vi "DAQ_AI_Open.vi"(0 "reference in":refnum<class "NI_DAQ.lvclass">, 5 "error in (no error)":errorcluster) -> (14 "reference out":refnum<class "NI_DAQ.lvclass">, 19 "error out":errorcluster)   [LabVIEW 2020, in "DAQ.lvlib" / "NI_DAQ.lvclass"]
uses:
  NI_DAQ.lvclass
panel:
  out "DAQ_AI_task_out":refnum<k21>
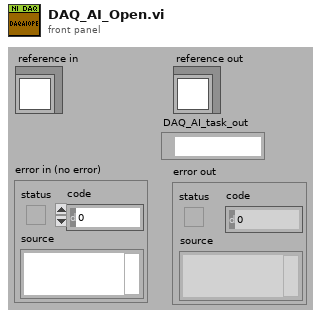
[diagram p1: front panel]
types:
  T1 = typedef "DAQ.lvlib/DAQ_Base.lvclass/DAQSettings.ctl" = cluster{"SampleSettings":T2, "AI_ChannelSettings":T3, "AO_ChannelSettings":T5, "Cnt_ChannelSettings":T6}
  T2 = typedef "DAQ.lvlib/DAQ_Base.lvclass/SampleSettings.ctl" = cluster{"samples per channel":i32, "SampleRate":dbl, "TansMaxLength":dbl, "ReadTimeOut":dbl, "时钟源":tag}
  T3 = typedef "DAQ.lvlib/DAQ_Base.lvclass/AI_ChannelSettings.ctl" = cluster{"AI_SettingsArry":cluster{"DeviceName":tag, "physical channels":tag, "AssignName":string, "输入信号类型":T4, "Max_value":dbl, "Min_value":dbl, "单位":i32, "shunt resistor location":i32, "external shunt resistor value":dbl, "标定系数":cluster{"Scale":dbl, "Offset":dbl}}[]}
  T4 = typedef "AI信号类型.ctl" = i32
  T5 = typedef "DAQ.lvlib/DAQ_Base.lvclass/AO_ChannelSettings.ctl" = cluster{"布尔":bool}
  T6 = typedef "DAQ.lvlib/DAQ_Base.lvclass/Cnt_ChannelSettings.ctl" = cluster{"Cnt_ChannelSettings":cluster{"类型":enum16{"Linear", "Rotate"}, "CounterNbr":tag, "AssignName":string, "单位":u16, "decoding type":u16, "PPR_DistancePerPulse":dbl, "Initial Position ":dbl, "z index enable":bool, "z index phase":i32, "source":tag}[]}
  T7 = typedef "DAQ.lvlib/NI_DAQ.lvclass/ObjectAttributesRef.ctl" = refnum<data-value>
  T8 = typedef "DAQ.lvlib/NI_DAQ.lvclass/ObjectAttributes.ctl" = cluster{"MyAttribute":dbl, "DAQ_AI_task_out":refnum<k21>, "counter_task_out":refnum<k21>[]}
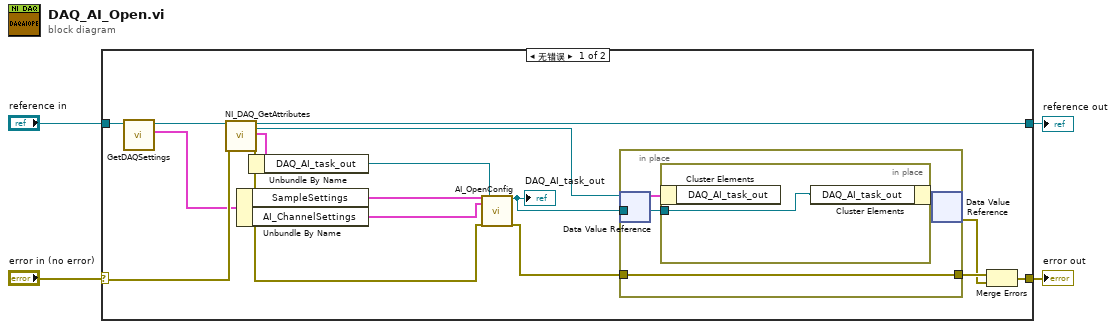
[diagram p0: block diagram]
diagram:
  n1 = case shown="无错误" "error in (no error)" {
    selector: "error in (no error)" -> [w18 w27]
    tunnel: [w20 w27] -> w3
    tunnel: [w19 w26] -> w1
    tunnel: "reference in" -> [w13 w26]
    frame No Error {
      n2 = call-dynamic "GetDAQSettings.vi"("reference in"=w13) -> ("DAQSettings"=w11:T1, "reference out"=w12:refnum<class "NI_DAQ.lvclass">)  [unwired: 8 in, 1 out]
      n3 = call "NI_DAQ_GetAttributes.vi"("reference in"=w12, "error in (no error)"=w18) -> ("reference out"=w19:refnum<class "NI_DAQ.lvclass">, "attributes ref"=w14:T7, "attributes"=w17:T8, "error out"=w9:errorcluster)  [unwired: 14 in]
      n4 = Unbundle By Name(w11) -> ("SampleSettings"=w10:T2, "AI_ChannelSettings"=w6:T3)
      n5 = Unbundle By Name(w17) -> ("DAQ_AI_task_out"=w5:refnum<k21>)
      n6 = call "AI_OpenConfig.vi"("SampleSettings"=w10, "AI_ChannelSettings"=w6, "error in"=w9, "DAQ_AI_task_out"=w5) -> ("DAQ_AI_task_out"=w7:refnum<k21>, "error out"=w8:errorcluster)  [unwired: 14 in]
      "DAQ_AI_task_out" <- w7
      n7 = in-place {
        in-place-border: w8 -> [w22]
        in-place-border: [w22] -> w16
        in-place-border: w7 -> [w21]
        n8 = in-place-dvr #1(w14) -> (w23:T8)  [unwired: 1 out]
        n9 = in-place {
          in-place-border: w21 -> [w25]
          n10 = in-place-cluster #2(w23) -> ()  [unwired: 1 out]
          n11 = in-place-cluster #2("DAQ_AI_task_out"=w25) -> (w24:T8)
        }
        n12 = in-place-dvr #1(w24) -> (w15:errorcluster)  [unwired: 1 out]
      }
      n13 = Merge Errors(w16, w15) -> (w20:errorcluster)
    }
    frame Error {
    }
  }
  "error out" <- w3
  "reference out" <- w1
